vi "pumonarytesting_auto_attempt2.vi"() -> ()   [LabVIEW 2014]
uses:
  <vilib>/vision/NI_Vision_Development_Module.lvlib
  <instrlib>/KD Scientific 2XX Series/KD Scientific 2XX Series.lvlib
panel:
  in  "Number of Cycles":i32
  in  "Min Pressure":dbl
  in  "Max Pressure":dbl
  out "Status":T1
  in  "stop 2":bool
  out "Delivered Volume":dbl
  out "Units":string
  in  "Baud Rate (9600)":u32(ring)=9600 items=["300"=300, "1200"=1200, "2400"=2400, "4800"=4800, "9600"=9600]
  in  "Withdrawal Settings":T2={"Flow Rate (5)"=5.0, "Volume (10)"=10.0, "Volume Units (ml)"=enum."milliliters (ml)", "Rate Units (ml/min.)"=enum."milliliters per minute (ml/min.)"} {"Volume (10)" format="%#.3g"}
  in  "Diameter (8.75 mm)":dbl=8.75
  in  "Infusion Settings":T2={"Flow Rate (5)"=5.0, "Volume (10)"=10.0, "Volume Units (ml)"=enum."milliliters (ml)", "Rate Units (ml/min.)"=enum."milliliters per minute (ml/min.)"}
  in  "Address (0)":i32 format="%0.0f"
  in  "error in (no error)":errorcluster
  in  "VISA resource name":refnum<visa-resource-name>="COM1"
  in  "stop 4":bool
  in  "stop":bool
  out "Image":T3(plugin-control)
  out "Particle Measurements (Pixels) (Particle Analysis 1)":dbl[][](array[numeric]) format="%.2f"
  out "subarray":dbl[](array[numeric])
  out "The diameter":dbl[](array[numeric])
  in  "stop (F)":bool
  out "Data from Transducer":dynamicdata(graph) caption="Voltage from Transducer V"
  out "Voltage from pressure transducer":dbl[](array[numeric])
  out "Pressure mm Hg":dbl[](graph)
  in  "Calibration factor":dbl[](array[numeric])
  in  "Zero Error":dbl[](array[numeric])
  out "pressure mm Hg":dbl[](array[numeric])
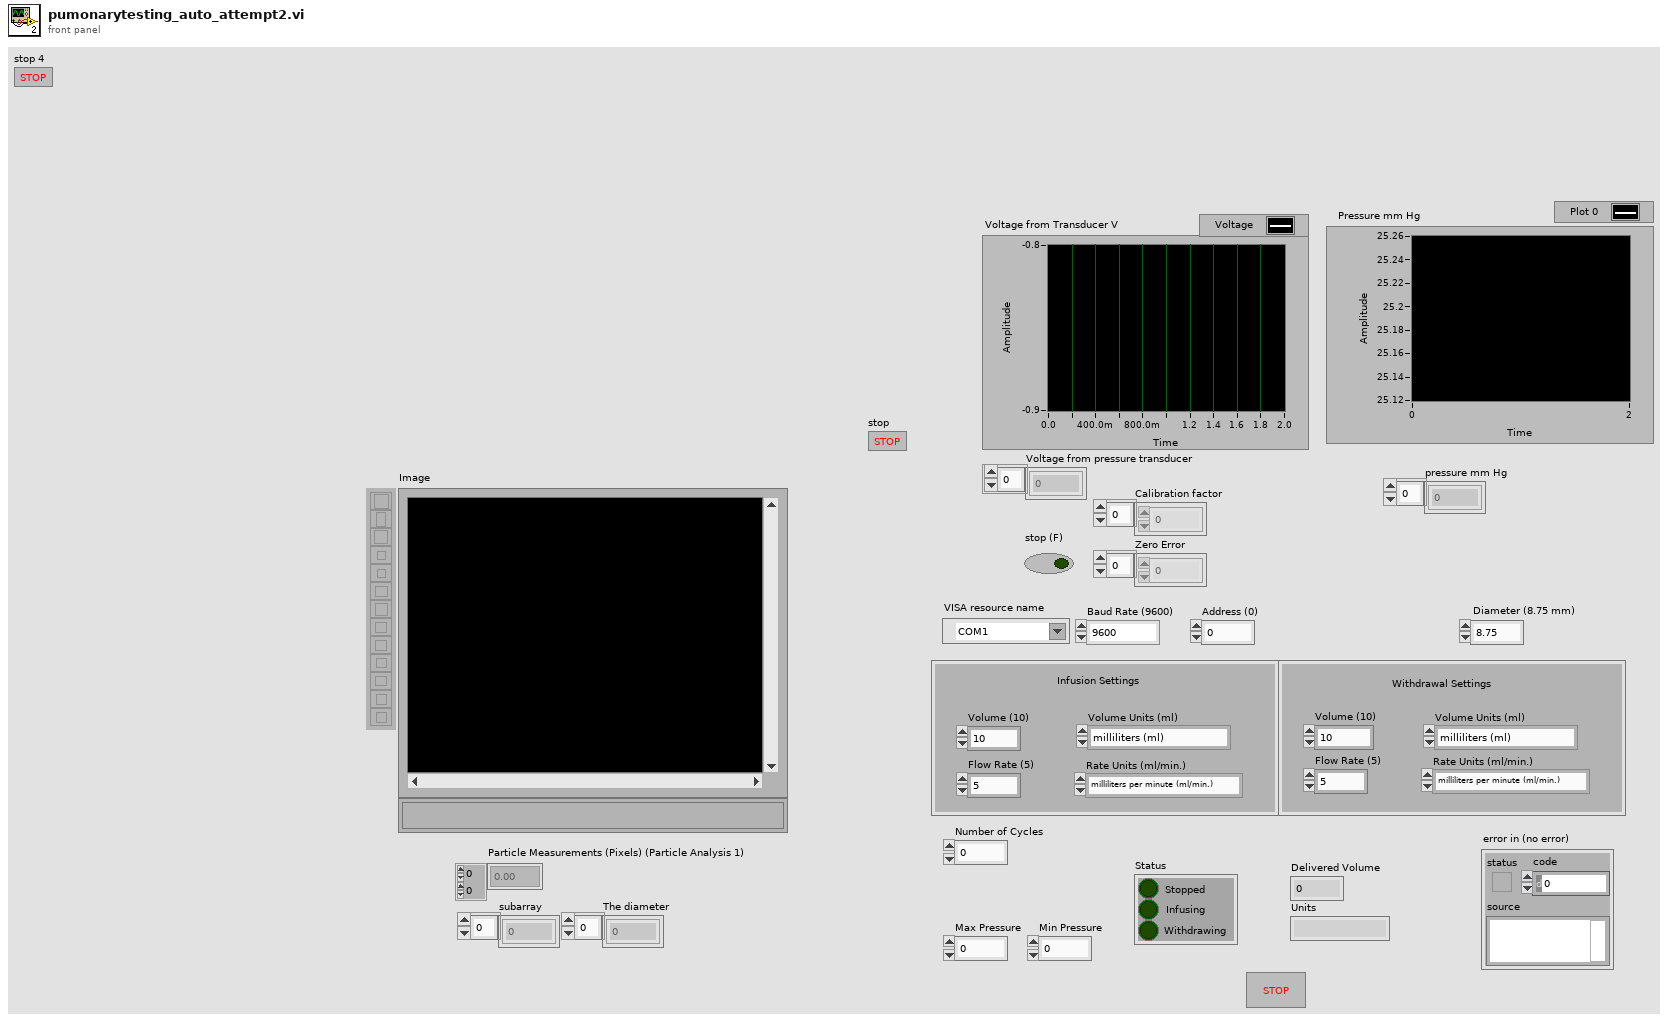
[diagram p1: front panel]
types:
  T1 = cluster{"Stopped":bool, "Infusing":bool, "Withdrawing":bool}
  T2 = cluster{"Flow Rate (5)":dbl, "Volume (10)":dbl, "Volume Units (ml)":enum16{"milliliters (ml)", "microliters (ul)"}, "Rate Units (ml/min.)":enum16{"milliliters per minute (ml/min.)", "milliliters per hour (ml/hr.)", "microliters per minute (ul/min.)", "microliters per hour (ul/hr.)"}}
  T3 = typedef "IMAQ Image.ctl" = refnum<image>
  T4 = typedef "Board Id" = u8
  T5 = typedef "ROI Descriptor" = cluster{"Global Rectangle":i32[], "Contours":cluster{"ID":enum32{"External", "Internal"}, "Type":u32, "Coordinates":i32[]}[]}
  T6 = enum16{"milliliters per minute (ml/min.)", "milliliters per hour (ml/hr.)", "microliters per minute (ul/min.)", "microliters per hour (ul/hr.)"}
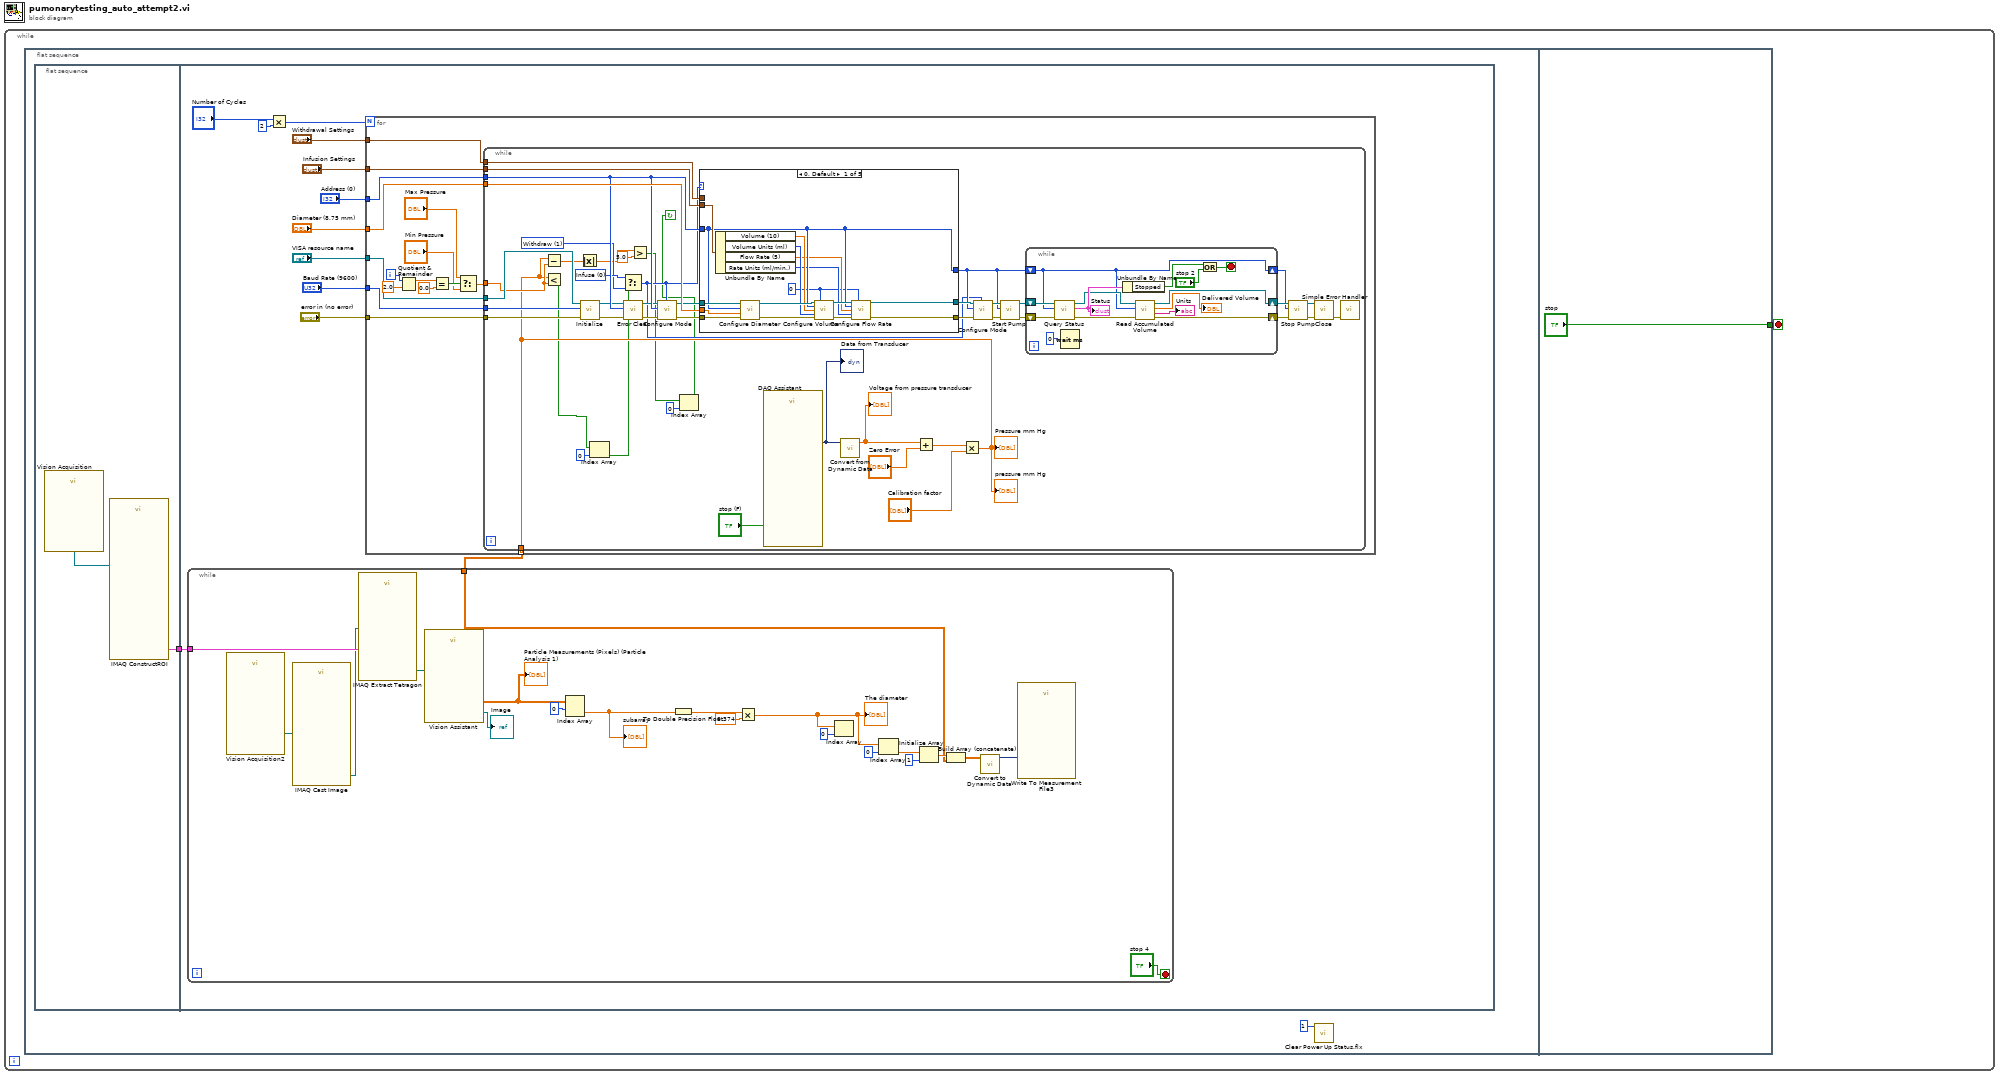
[diagram p0: block diagram]
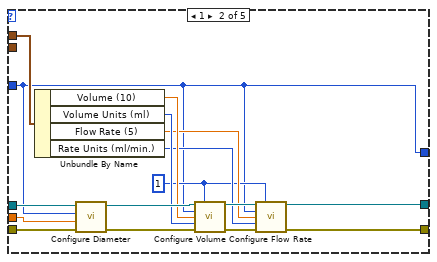
[diagram p2: hidden frame]
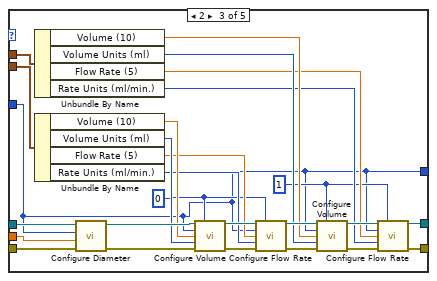
[diagram p3: hidden frame]
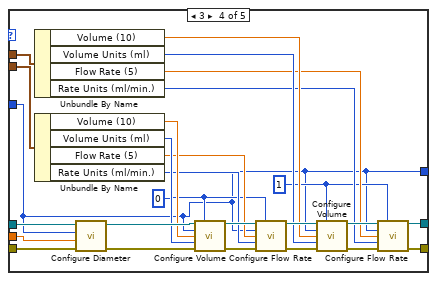
[diagram p4: hidden frame]
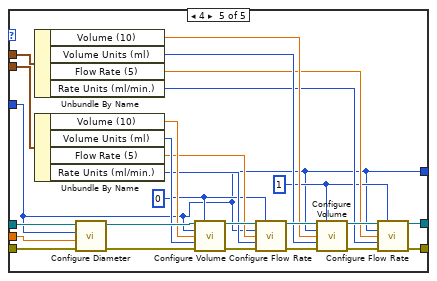
[diagram p5: hidden frame]
diagram:
  n1 = while {
    stop <- w1 stop-if-true
    n2 = flat-sequence {
      tunnel: ["stop"] -> w1
      frame #0 {
        n3 = flat-sequence {
          tunnel: [w4] -> w3
          tunnel: w3 -> [w17]
          frame #0 {
            n4 = call "Vision Acquisition"() -> ("Image Out"=w5:T3)  [unwired: 26 in, 1 out]
            n5 = call "IMAQ ConstructROI"("Image"=w5) -> ("ROI Descriptor Out"=w4:T5)  [unwired: 7 in, 3 out]
          }
          frame #1 {
            n6 = Multiply(x="Number of Cycles", y=2) -> (x*y=w16:i32)
            n7 = for {
              N: w16 -> [_]
              tunnel: "VISA resource name" -> [w33]
              tunnel: "error in (no error)" -> [w32]
              tunnel: "Infusion Settings" -> [w31]
              tunnel: "Withdrawal Settings" -> [w30]
              tunnel: "Diameter (8.75 mm)" -> [w29]
              tunnel: "Baud Rate (9600)" -> [w28]
              tunnel: "Address (0)" -> [w27]
              tunnel: [w18] -> w6 mode=indexing
              i -> [w25]
              n8 = Quotient & Remainder(x=w25, y=2.0) -> (x-y*floor(x/y)=w23:dbl)  [unwired: 1 out]
              n9 = Equal?(x=w23, y=0.0) -> (x = y?=w22:bool)
              n10 = Select(t="Max Pressure", s=w22, f="Min Pressure") -> (s? t:f=w19:dbl)
              n11 = while {
                tunnel: w33 -> [w79]
                tunnel: w32 -> [w78]
                tunnel: w31 -> [w77]
                tunnel: w30 -> [w76]
                tunnel: w29 -> [w75]
                tunnel: w28 -> [w74]
                tunnel: w27 -> [w73]
                tunnel: w19 -> [w50]
                tunnel: [w40] -> w18
                stop <- w34 continue-if-true
                w52 = u16 1 items=["Withdraw"=1]
                w53 = u16 0 items=["Infuse"] ("Mode (infuse)")
                n12 = call <instrlib>:"Initialize.vi"("error in (no error)"=w78, "Baud Rate (9600)"=w74, "VISA resource name"=w79) -> ("error out"=w55:errorcluster, "VISA resource name out"=w54:refnum<visa-resource-name>)  [unwired: 7 in]
                n13 = call <instrlib>:"Error Clear.vi"("error in (no error)"=w55, "Address (0)"=w73, "VISA resource name"=w54) -> ("error out"=w56:errorcluster, "VISA resource name out"=w57:refnum<visa-resource-name>)  [unwired: 6 in, 1 out]
                n14 = call "DAQ Assistant"("stop (F)"="stop (F)") -> ("data"=w41:dynamicdata)  [unwired: 15 in, 3 out]
                "Data from Transducer" <- w41
                n15 = call "Convert from Dynamic Data"("Dynamic Data Type"=w41) -> ("Array"=w44:dbl[])  [unwired: 3 in]
                "Voltage from pressure transducer" <- w44
                n16 = Add(x=w44, y="Zero Error") -> (x+y=w42:dbl[])
                n17 = Multiply(x=w42, y="Calibration factor") -> (x*y=w40:dbl[])
                "Pressure mm Hg" <- w40
                "pressure mm Hg" <- w40
                n18 = Subtract(x=w40, y=w50) -> (x-y=w49:dbl[])
                n19 = Less?(x=w40, y=w50) -> (x < y?=w39:bool[])
                n20 = Absolute Value(x=w49) -> (abs(x)=w48:dbl[])
                n21 = Index Array(array=w39, index=0) -> (element=w37:bool)
                n22 = Select(t=w53, s=w37, f=w52) -> (s? t:f=w51:u16)
                n23 = Greater?(x=w48, y=5.0) -> (0:w36:bool[])
                n24 = call <instrlib>:"Configure Mode.vi"("Mode (infuse)"=w51, "error in (no error)"=w56, "Address (0)"=w73, "VISA resource name"=w57) -> ("error out"=w59:errorcluster, "VISA resource name out"=w58:refnum<visa-resource-name>)  [unwired: 6 in]
                n25 = Index Array(array=w36, index=0) -> (element=w34:bool)
                n26 = case shown="0, Default" w51 {
                  tunnel: w77 -> [w89 _ w137 w163 w189]
                  tunnel: w76 -> [_ w111 w136 w162 w188]
                  tunnel: w58 -> [w95 w110 w135 w161 w187]
                  tunnel: w59 -> [w94 w106 w134 w160 w186]
                  tunnel: w75 -> [w88 w102 w117 w143 w169]
                  tunnel: [w87 w96 w112 w138 w164] -> w60
                  tunnel: w73 -> [w87 w96 w112 w138 w164]
                  tunnel: [w82 w107 w114 w140 w166] -> w64
                  tunnel: [w81 w103 w113 w139 w165] -> w63
                  frame 0, Default {
                    w80 = 0
                    n27 = Unbundle By Name(w89) -> ("Volume (10)"=w86:dbl, "Volume Units (ml)"=w85:enum16{"milliliters (ml)", "microliters (ul)"}, "Flow Rate (5)"=w84:dbl, "Rate Units (ml/min.)"=w83:T6)
                    n28 = call <instrlib>:"Configure Diameter.vi"("error in (no error)"=w94, "Diameter (8.75 mm)"=w88, "Address (0)"=w87, "VISA resource name"=w95) -> ("error out"=w92:errorcluster, "VISA resource name out"=w93:refnum<visa-resource-name>)  [unwired: 6 in]
                    n29 = call <instrlib>:"Configure Volume.vi"("VISA resource name"=w93, "Mode (infuse)"=w80, "Address (0)"=w87, "Volume (100)"=w86, "Units (0: milliliters)"=w85, "error in (no error)"=w92) -> ("VISA resource name out"=w91:refnum<visa-resource-name>, "error out"=w90:errorcluster)  [unwired: 8 in]
                    n30 = call <instrlib>:"Configure Flow Rate.vi"("VISA resource name"=w91, "Mode (infuse)"=w80, "Address (0)"=w87, "Flow Rate (5)"=w84, "Units (0: milliliters per minute)"=w83, "error in (no error)"=w90) -> ("VISA resource name out"=w82:refnum<visa-resource-name>, "error out"=w81:errorcluster)  [unwired: 8 in]
                  }
                  frame 1 {
                    w97 = 1
                    n31 = Unbundle By Name(w111) -> ("Volume (10)"=w101:dbl, "Volume Units (ml)"=w100:enum16{"milliliters (ml)", "microliters (ul)"}, "Flow Rate (5)"=w99:dbl, "Rate Units (ml/min.)"=w98:T6)
                    n32 = call <instrlib>:"Configure Diameter.vi"("error in (no error)"=w106, "Diameter (8.75 mm)"=w102, "Address (0)"=w96, "VISA resource name"=w110) -> ("error out"=w105:errorcluster, "VISA resource name out"=w109:refnum<visa-resource-name>)  [unwired: 6 in]
                    n33 = call <instrlib>:"Configure Volume.vi"("VISA resource name"=w109, "Mode (infuse)"=w97, "Address (0)"=w96, "Volume (100)"=w101, "Units (0: milliliters)"=w100, "error in (no error)"=w105) -> ("VISA resource name out"=w108:refnum<visa-resource-name>, "error out"=w104:errorcluster)  [unwired: 8 in]
                    n34 = call <instrlib>:"Configure Flow Rate.vi"("VISA resource name"=w108, "Mode (infuse)"=w97, "Address (0)"=w96, "Flow Rate (5)"=w99, "Units (0: milliliters per minute)"=w98, "error in (no error)"=w104) -> ("VISA resource name out"=w107:refnum<visa-resource-name>, "error out"=w103:errorcluster)  [unwired: 8 in]
                  }
                  frame 2 {
                    w115 = 1
                    w116 = 0
                    n35 = Unbundle By Name(w136) -> ("Volume (10)"=w121:dbl, "Volume Units (ml)"=w120:enum16{"milliliters (ml)", "microliters (ul)"}, "Flow Rate (5)"=w119:dbl, "Rate Units (ml/min.)"=w118:T6)
                    n36 = Unbundle By Name(w137) -> ("Volume (10)"=w125:dbl, "Volume Units (ml)"=w124:enum16{"milliliters (ml)", "microliters (ul)"}, "Flow Rate (5)"=w123:dbl, "Rate Units (ml/min.)"=w122:T6)
                    n37 = call <instrlib>:"Configure Diameter.vi"("error in (no error)"=w134, "Diameter (8.75 mm)"=w117, "Address (0)"=w112, "VISA resource name"=w135) -> ("error out"=w129:errorcluster, "VISA resource name out"=w133:refnum<visa-resource-name>)  [unwired: 6 in]
                    n38 = call <instrlib>:"Configure Volume.vi"("VISA resource name"=w133, "Mode (infuse)"=w116, "Address (0)"=w112, "Volume (100)"=w125, "Units (0: milliliters)"=w124, "error in (no error)"=w129) -> ("VISA resource name out"=w132:refnum<visa-resource-name>, "error out"=w128:errorcluster)  [unwired: 8 in]
                    n39 = call <instrlib>:"Configure Flow Rate.vi"("VISA resource name"=w132, "Mode (infuse)"=w116, "Address (0)"=w112, "Flow Rate (5)"=w123, "Units (0: milliliters per minute)"=w122, "error in (no error)"=w128) -> ("VISA resource name out"=w131:refnum<visa-resource-name>, "error out"=w127:errorcluster)  [unwired: 8 in]
                    n40 = call <instrlib>:"Configure Volume.vi"("VISA resource name"=w131, "Mode (infuse)"=w115, "Address (0)"=w112, "Volume (100)"=w121, "Units (0: milliliters)"=w120, "error in (no error)"=w127) -> ("VISA resource name out"=w130:refnum<visa-resource-name>, "error out"=w126:errorcluster)  [unwired: 8 in]
                    n41 = call <instrlib>:"Configure Flow Rate.vi"("VISA resource name"=w130, "Mode (infuse)"=w115, "Address (0)"=w112, "Flow Rate (5)"=w119, "Units (0: milliliters per minute)"=w118, "error in (no error)"=w126) -> ("VISA resource name out"=w114:refnum<visa-resource-name>, "error out"=w113:errorcluster)  [unwired: 8 in]
                  }
                  frame 3 {
                    w141 = 1
                    w142 = 0
                    n42 = Unbundle By Name(w162) -> ("Volume (10)"=w147:dbl, "Volume Units (ml)"=w146:enum16{"milliliters (ml)", "microliters (ul)"}, "Flow Rate (5)"=w145:dbl, "Rate Units (ml/min.)"=w144:T6)
                    n43 = Unbundle By Name(w163) -> ("Volume (10)"=w151:dbl, "Volume Units (ml)"=w150:enum16{"milliliters (ml)", "microliters (ul)"}, "Flow Rate (5)"=w149:dbl, "Rate Units (ml/min.)"=w148:T6)
                    n44 = call <instrlib>:"Configure Diameter.vi"("error in (no error)"=w160, "Diameter (8.75 mm)"=w143, "Address (0)"=w138, "VISA resource name"=w161) -> ("error out"=w155:errorcluster, "VISA resource name out"=w159:refnum<visa-resource-name>)  [unwired: 6 in]
                    n45 = call <instrlib>:"Configure Volume.vi"("VISA resource name"=w159, "Mode (infuse)"=w142, "Address (0)"=w138, "Volume (100)"=w151, "Units (0: milliliters)"=w150, "error in (no error)"=w155) -> ("VISA resource name out"=w158:refnum<visa-resource-name>, "error out"=w154:errorcluster)  [unwired: 8 in]
                    n46 = call <instrlib>:"Configure Flow Rate.vi"("VISA resource name"=w158, "Mode (infuse)"=w142, "Address (0)"=w138, "Flow Rate (5)"=w149, "Units (0: milliliters per minute)"=w148, "error in (no error)"=w154) -> ("VISA resource name out"=w157:refnum<visa-resource-name>, "error out"=w153:errorcluster)  [unwired: 8 in]
                    n47 = call <instrlib>:"Configure Volume.vi"("VISA resource name"=w157, "Mode (infuse)"=w141, "Address (0)"=w138, "Volume (100)"=w147, "Units (0: milliliters)"=w146, "error in (no error)"=w153) -> ("VISA resource name out"=w156:refnum<visa-resource-name>, "error out"=w152:errorcluster)  [unwired: 8 in]
                    n48 = call <instrlib>:"Configure Flow Rate.vi"("VISA resource name"=w156, "Mode (infuse)"=w141, "Address (0)"=w138, "Flow Rate (5)"=w145, "Units (0: milliliters per minute)"=w144, "error in (no error)"=w152) -> ("VISA resource name out"=w140:refnum<visa-resource-name>, "error out"=w139:errorcluster)  [unwired: 8 in]
                  }
                  frame 4 {
                    w167 = 1
                    w168 = 0
                    n49 = Unbundle By Name(w188) -> ("Volume (10)"=w173:dbl, "Volume Units (ml)"=w172:enum16{"milliliters (ml)", "microliters (ul)"}, "Flow Rate (5)"=w171:dbl, "Rate Units (ml/min.)"=w170:T6)
                    n50 = Unbundle By Name(w189) -> ("Volume (10)"=w177:dbl, "Volume Units (ml)"=w176:enum16{"milliliters (ml)", "microliters (ul)"}, "Flow Rate (5)"=w175:dbl, "Rate Units (ml/min.)"=w174:T6)
                    n51 = call <instrlib>:"Configure Diameter.vi"("error in (no error)"=w186, "Diameter (8.75 mm)"=w169, "Address (0)"=w164, "VISA resource name"=w187) -> ("error out"=w181:errorcluster, "VISA resource name out"=w185:refnum<visa-resource-name>)  [unwired: 6 in]
                    n52 = call <instrlib>:"Configure Volume.vi"("VISA resource name"=w185, "Mode (infuse)"=w168, "Address (0)"=w164, "Volume (100)"=w177, "Units (0: milliliters)"=w176, "error in (no error)"=w181) -> ("VISA resource name out"=w184:refnum<visa-resource-name>, "error out"=w180:errorcluster)  [unwired: 8 in]
                    n53 = call <instrlib>:"Configure Flow Rate.vi"("VISA resource name"=w184, "Mode (infuse)"=w168, "Address (0)"=w164, "Flow Rate (5)"=w175, "Units (0: milliliters per minute)"=w174, "error in (no error)"=w180) -> ("VISA resource name out"=w183:refnum<visa-resource-name>, "error out"=w179:errorcluster)  [unwired: 8 in]
                    n54 = call <instrlib>:"Configure Volume.vi"("VISA resource name"=w183, "Mode (infuse)"=w167, "Address (0)"=w164, "Volume (100)"=w173, "Units (0: milliliters)"=w172, "error in (no error)"=w179) -> ("VISA resource name out"=w182:refnum<visa-resource-name>, "error out"=w178:errorcluster)  [unwired: 8 in]
                    n55 = call <instrlib>:"Configure Flow Rate.vi"("VISA resource name"=w182, "Mode (infuse)"=w167, "Address (0)"=w164, "Flow Rate (5)"=w171, "Units (0: milliliters per minute)"=w170, "error in (no error)"=w178) -> ("VISA resource name out"=w166:refnum<visa-resource-name>, "error out"=w165:errorcluster)  [unwired: 8 in]
                  }
                }
                n56 = call <instrlib>:"Configure Mode.vi"("Mode (infuse)"=w51, "error in (no error)"=w63, "Address (0)"=w60, "VISA resource name"=w64) -> ("error out"=w61:errorcluster, "VISA resource name out"=w62:refnum<visa-resource-name>)  [unwired: 6 in]
                n57 = call <instrlib>:"Start Pump.vi"("error in (no error)"=w61, "Address (0)"=w60, "VISA resource name"=w62) -> ("error out"=w71:errorcluster, "VISA resource name out"=w72:refnum<visa-resource-name>)  [unwired: 7 in]
                n58 = while {
                  shift-right: [w192] -> w68
                  shift-left: w60 -> [w192]
                  shift-right: [w194] -> w70
                  shift-left: w72 -> [w200]
                  shift-right: [w193] -> w69
                  shift-left: w71 -> [w201]
                  stop <- w198 stop-if-true
                  n59 = call <instrlib>:"Query Status.vi"("error in (no error)"=w201, "Address (0)"=w192, "VISA resource name"=w200) -> ("error out"=w203:errorcluster, "Status"=w199:T1, "VISA resource name out"=w195:refnum<visa-resource-name>)  [unwired: 6 in]
                  "Status" <- w199
                  n60 = Wait (ms)(milliseconds to wait=u32 0) -> ()  [unwired: 1 out]
                  n61 = Unbundle By Name(w199) -> ("Stopped"=w197:bool)
                  n62 = call <instrlib>:"Read Accumulated Volume.vi"("error in (no error)"=w203, "Address (0)"=w192, "VISA resource name"=w195) -> ("error out"=w193:errorcluster, "Units"=→"Units":string, "Delivered Volume"=→"Delivered Volume":dbl, "VISA resource name out"=w194:refnum<visa-resource-name>)  [unwired: 5 in]
                  n63 = Or(x=w197, y="stop 2") -> (x .or. y?=w198:bool)
                }
                n64 = call <instrlib>:"Stop Pump.vi"("error in (no error)"=w69, "Address (0)"=w68, "VISA resource name"=w70) -> ("error out"=w66:errorcluster, "VISA resource name out"=w65:refnum<visa-resource-name>)  [unwired: 7 in]
                n65 = call <instrlib>:"Close.vi"("error in (no error)"=w66, "VISA resource name"=w65) -> ("error out"=w67:errorcluster)  [unwired: 9 in]
                n66 = call <vilib>:"Simple Error Handler.vi"("error in (no error)"=w67) -> ()  [unwired: 4 in, 5 out]
              }
            }
            n67 = while {
              tunnel: w17 -> [w223]
              tunnel: w6 -> [w204]
              stop <- "stop 4" stop-if-true
              n68 = call "Vision Acquisition2"() -> ("Image Out"=w213:T3)  [unwired: 25 in, 2 out]
              n69 = call "IMAQ Cast Image"("Image Src"=w213) -> ("Image Dst Out"=w220:T3)  [unwired: 9 in, 1 out]
              n70 = call-poly "IMAQ Extract Tetragon"("ROI Descriptor"=w223, "Image Src"=w220) -> ("Image Dst Out"=w221:T3)  [unwired: 8 in, 1 out]
              n71 = call "Vision Assistant"("Image In"=w221) -> ("Image Out"=→"Image":T3, "Particle Measurements (Pixels) (Particle Analysis 1)"=w219:dbl[][])  [unwired: 23 in, 2 out]
              "Particle Measurements (Pixels) (Particle Analysis 1)" <- w219
              n72 = Index Array(array=w219, index (row)=0) -> (element=w217:dbl[])  [unwired: 1 in]
              "subarray" <- w217
              n73 = To Double Precision Float(number=w217) -> (double precision float=w216:dbl[])
              n74 = Multiply(x=w216, y=0.374) -> (x*y=w210:dbl[])
              "The diameter" <- w210
              n75 = Index Array(array=w210, index=0) -> ()  [unwired: 1 out]
              n76 = Index Array(array=w210, index=0) -> (element=w209:dbl)
              n77 = Initialize Array(w209, 1 ("dimension size")) -> (w207:dbl[])
              n78 = Build Array (concatenate)(w207, w204) -> (w206:dbl[][])
              n79 = call "Convert to Dynamic Data"("2D Array"=w206) -> ("Dynamic Data Type"=w205:dynamicdata)  [unwired: 3 in]
              n80 = call "Write To Measurement File3"("Signals"=w205) -> ()  [unwired: 16 in, 3 out]
            }
          }
        }
        n81 = call <vilib>:"Clear Power Up Status.flx"("Board ID"=T4 1) -> ()  [unwired: 6 in, 2 out]
      }
      frame #1 {
      }
    }
  }
